vi "波形.vi"() -> ()   [LabVIEW 2015]
panel:
  out "波形图3":cluster{dbl[]}[](graph)
  out "波形图2":dbl[][](graph)
  out "波形图1":dbl[](graph)
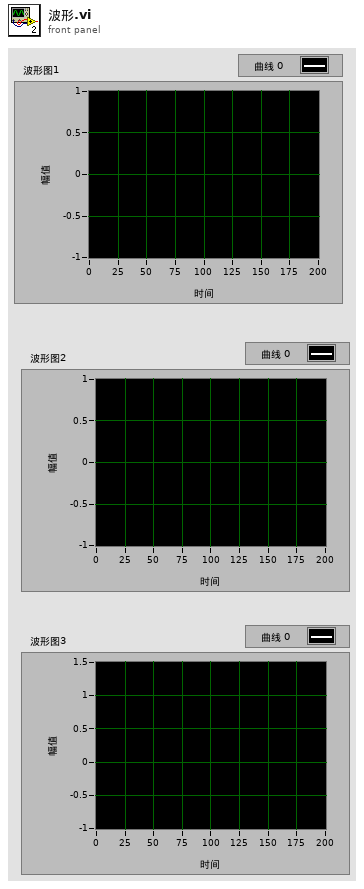
[diagram p1: front panel]
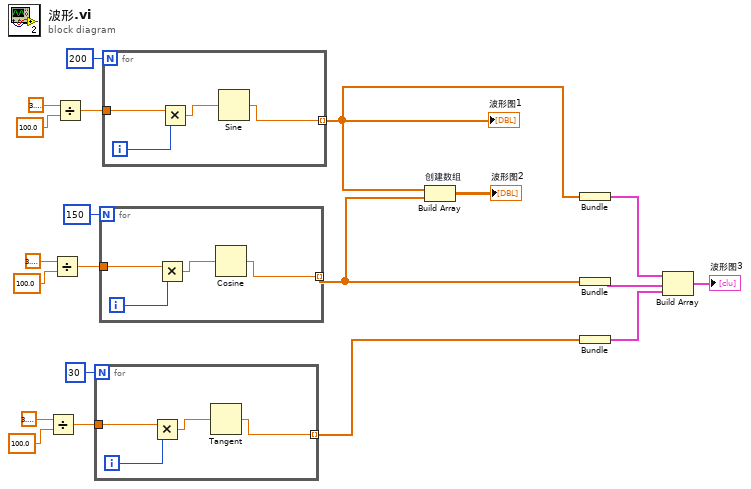
[diagram p0: block diagram]
diagram:
  n1 = Divide(x=3.141592653589793, y=100.0) -> (x/y=w8:dbl)
  n2 = Divide(x=3.141592653589793, y=100.0) -> (x/y=w16:dbl)
  n3 = Divide(x=3.141592653589793, y=100.0) -> (x/y=w17:dbl)
  n4 = for {
    N: 30 -> [_]
    tunnel: w8 -> [w24]
    tunnel: [w21] -> w1 mode=indexing
    i -> [w23]
    n5 = Multiply(x=w24, y=w23) -> (x*y=w22:dbl)
    n6 = Tangent(1:w22) -> (0:w21:dbl)
  }
  n7 = for {
    N: 150 -> [_]
    tunnel: w16 -> [w28]
    tunnel: [w25] -> w6 mode=indexing
    i -> [w27]
    n8 = Multiply(x=w28, y=w27) -> (x*y=w26:dbl)
    n9 = Cosine(x=w26) -> (cos(x)=w25:dbl)
  }
  n10 = for {
    N: 200 -> [_]
    tunnel: w17 -> [w32]
    tunnel: [w29] -> w7 mode=indexing
    i -> [w31]
    n11 = Multiply(x=w32, y=w31) -> (x*y=w30:dbl)
    n12 = Sine(x=w30) -> (sin(x)=w29:dbl)
  }
  "波形图1" <- w7
  n13 = Build Array "创建数组"(w7, w6) -> (→"波形图2":dbl[][])
  n14 = Bundle(w7) -> (w5:cluster{dbl[]})  [unwired: 1 in]
  n15 = Bundle(w6) -> (w4:cluster{dbl[]})  [unwired: 1 in]
  n16 = Bundle(w1) -> (w2:cluster{dbl[]})  [unwired: 1 in]
  n17 = Build Array(w5, w4, w2) -> (→"波形图3":cluster{dbl[]}[])
